vi "SSV_target_nocatch_frequency.vi"() -> ()   [LabVIEW 2014]
uses:
  <vilib>/userdefined/High Color/IMAQdx.ctl
  <vilib>/vision/driver/IMAQdx.llb/IMAQdx Acquisition Mode.ctl
  <vilib>/myRIO/Instrument Drivers/Onboard IO/PWM/typedefs/PWM Reference.ctl
  <vilib>/myRIO/Common/Instrument Driver Framework/Utilities/typedefs/myRIO Generic Hardware Reference.ctl
  <vilib>/myRIO/Common/Instrument Driver Framework/Utilities/typedefs/Hardware Version Enum.ctl
  <vilib>/myRIO/Common/Instrument Driver Framework/Utilities/typedefs/myRIO v1.0 Reference.ctl
  <vilib>/myRIO/Common/Instrument Driver Framework/Utilities/typedefs/Generic FPGA Reference.ctl
  <vilib>/myRIO/Common/Instrument Driver Framework/myRIO v1.0/PWM/typedefs/PWM Channels Enum.ctl
  <vilib>/myRIO/Instrument Drivers/Onboard IO/PWM/typedefs/PWM Configuration.ctl
  <vilib>/userdefined/High Color/nirio_resource_hc.ctl
  <vilib>/myRIO/Instrument Drivers/Onboard IO/DIO/typedefs/DIO Reference.ctl
  <vilib>/myRIO/Common/Instrument Driver Framework/myRIO v1.0/DIO/typedefs/DIO Channels List.ctl
  <vilib>/myRIO/Common/Instrument Driver Framework/myRIO v1.0/DIO/typedefs/DIO Channels Enum.ctl
  <vilib>/vision/driver/IMAQdx.llb/IMAQdx Buffer Number Mode.ctl
  <vilib>/myRIO/Common/Instrument Driver Framework/myRIO v1.0/PWM/vis/myRIO v1.1 Open PWM.vi
  <vilib>/myRIO/Common/Instrument Driver Framework/myRIO v1.0/DIO/vis/myRIO v1.1 Open DIO.vi
  <vilib>/myRIO/Common/Instrument Driver Framework/Utilities/vis/Is FPGA Ref Available.vi
  <vilib>/myRIO/Instrument Drivers/Onboard IO/DIO/vis/Read.vi
  <vilib>/Analysis/baseanly.llb/Mean (DBL).vi
  <vilib>/myRIO/Common/Instrument Driver Framework/Utilities/vis/Validate Channels.vi
  <vilib>/myRIO/Common/Instrument Driver Framework/myRIO v1.0/PWM/vis/myRIO v1.0 Reserve PWM.vi
  <vilib>/myRIO/Common/Instrument Driver Framework/myRIO v1.0/DIO/vis/myRIO v1.0 Reserve DIO.vi
  <vilib>/myRIO/Common/Instrument Driver Framework/myRIO v1.0/DIO/vis/myRIO v1.0 Close DIO.vi
  <vilib>/myRIO/Common/Instrument Driver Framework/myRIO v1.0/PWM/vis/myRIO v1.0 Close PWM.vi
  <vilib>/myRIO/Common/Instrument Driver Framework/myRIO v1.0/PWM/vis/myRIO v1.0 Build MUX Configuration PWM.vi
  <vilib>/myRIO/Common/Instrument Driver Framework/myRIO v1.0/Resource Manager/vis/myRIO v1.0 Reserve Channel List.vi
  <vilib>/myRIO/Common/Instrument Driver Framework/myRIO v1.0/DIO/vis/myRIO v1.0 Build MUX Configuration DIO.vi
  <vilib>/myRIO/Common/Instrument Driver Framework/myRIO v1.0/DIO/vis/myRIO v1.0 Unreserve DIO.vi
  <vilib>/myRIO/Common/Instrument Driver Framework/myRIO v1.0/PWM/vis/myRIO v1.0 Unreserve PWM.vi
  <vilib>/myRIO/Common/Instrument Driver Framework/myRIO v1.0/Resource Manager/vis/myRIO v1.0 Create Configuration List.vi
  <vilib>/myRIO/Common/Instrument Driver Framework/myRIO v1.0/Resource Manager/vis/myRIO v1.0 Reserve Channel.vi
  <vilib>/myRIO/Common/Instrument Driver Framework/myRIO v1.0/Resource Manager/vis/myRIO v1.0 Unreserve Channel.vi
  <vilib>/myRIO/Common/Instrument Driver Framework/myRIO v1.0/Resource Manager/vis/myRIO v1.0 Unreserve Channel List.vi
  <vilib>/myRIO/Common/Instrument Driver Framework/myRIO v1.0/Resource Manager/vis/myRIO v1.0 Build Mutex Name.vi
  <vilib>/Utility/VariantDataType/GetNumericInfo.vi
  <vilib>/Utility/error.llb/Error Cluster From Error Code.vi
  <vilib>/myRIO/Common/Instrument Driver Framework/myRIO v1.0/myRIO v1.1 Open.vi
  <vilib>/myRIO/Common/Instrument Driver Framework/Utilities/vis/IO Manager.vi
  <vilib>/myRIO/Common/Instrument Driver Framework/Utilities/vis/Configuration Manager.vi
  <vilib>/myRIO/Common/Instrument Driver Framework/myRIO v1.0/Resource Manager/vis/myRIO v1.0 Configure IO.vi
  <vilib>/myRIO/Common/Instrument Driver Framework/myRIO v1.0/myRIO v1.0 Close.vi
  <vilib>/myRIO/Common/Instrument Driver Framework/myRIO v1.0/DIO/vis/myRIO v1.0 Write DIO.vi
  <vilib>/myRIO/Common/Instrument Driver Framework/myRIO v1.0/PWM/vis/myRIO v1.0 Write PWM.vi
  <vilib>/myRIO/Common/Instrument Driver Framework/myRIO v1.0/DIO/vis/myRIO v1.0 Read DIO.vi
  <vilib>/myRIO/Common/Instrument Driver Framework/myRIO v1.0/DIO/vis/myRIO v1.0 Shutdown DIO.vi
  <vilib>/myRIO/Common/Instrument Driver Framework/myRIO v1.0/PWM/vis/myRIO v1.0 Shutdown PWM.vi
  <vilib>/myRIO/Instrument Drivers/Onboard IO/DIO/vis/myRIO DIO Open.xnode
  <vilib>/myRIO/Instrument Drivers/Onboard IO/PWM/vis/myRIO PWM Open.xnode
  <vilib>/myRIO/Express VI/Onboard Devices/LED/LED Express VI.xnode
  <vilib>/myRIO/Express VI/Onboard Devices/Button/Button Express VI.xnode
  <vilib>/vision/driver/NI_Vision_Acquisition_Software.lvlib
  <vilib>/vision/NI_Vision_Development_Module.lvlib
  <vilib>/Analysis/NI_AALBase.lvlib
  <resource>/objmgr/imaqdx.rc
  <vilib>/myRIO/Instrument Drivers/Onboard IO/DIO/DIO.lvlib
  <vilib>/myRIO/Instrument Drivers/Onboard IO/PWM/PWM.lvlib
panel:
  in  "V":cluster{dbl, dbl}(slide)={0.0, 2.8282828282828283} scale=0.0..255.0
  in  "S":cluster{dbl, dbl}(slide)={0.0, 2.8282828282828283} scale=0.0..255.0
  in  "H":cluster{dbl, dbl}(slide)={0.0, 2.8282828282828283} scale=0.0..255.0
  out "PWM Error":errorcluster
  out "Array 5":bool[](array[boolean])
  out "Array 4":bool[](array[boolean])
  out "Array 3":bool[](array[boolean])
  out "Array 2":bool[](array[boolean])
  out "Motors":bool[](array[boolean])
  in  "Min Period (ms)":dbl=500.0 format="%#_13g"
  in  "Max Period (ms)":dbl=500.0 format="%#_13g"
  out "y":dbl
  out "x":dbl
  out "Tracking Image":T1(plugin-control)
  out "Distance (in)":dbl
  in  "Diameter of Ball (in)":dbl
  out "DIO Error":errorcluster
  in  "Max Distance (in)":dbl=500.0 format="%#_13g"
  out "Camera Error":errorcluster
  out "FPS":dbl
  out "Original Image":T1(plugin-control)
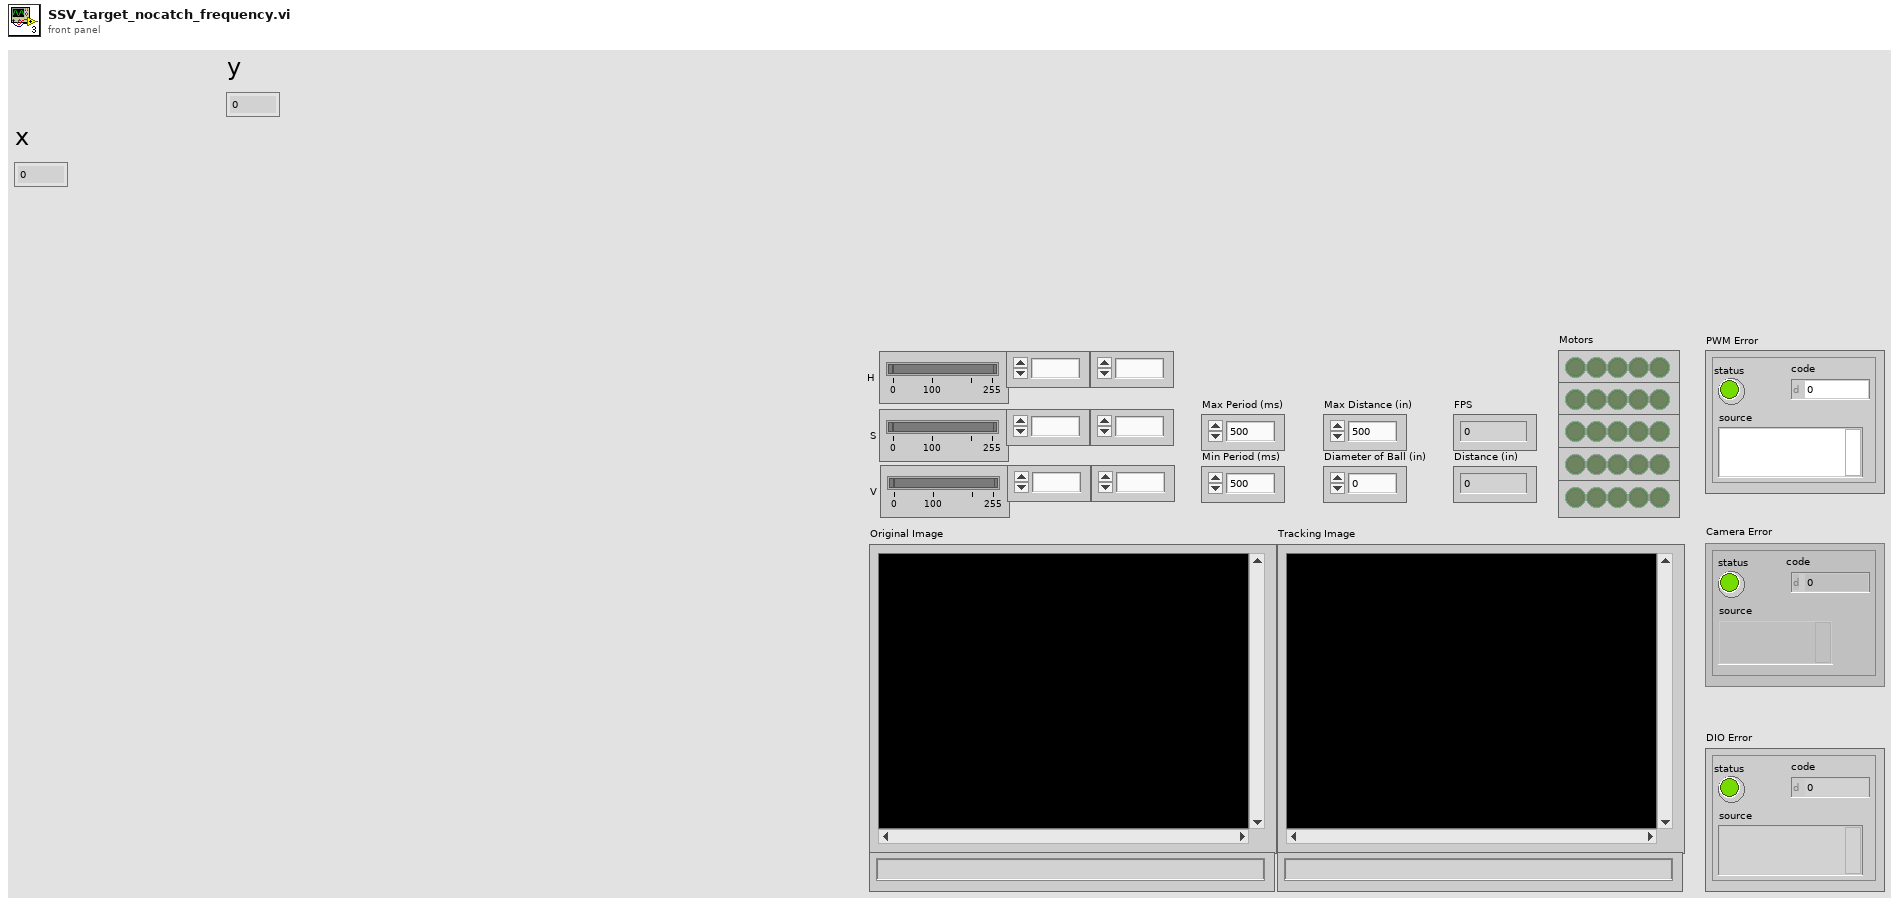
[diagram p1: front panel]
types:
  T1 = typedef "IMAQ Image.ctl" = refnum<image>
  T2 = typedef "NI_Vision_Acquisition_Software.lvlib/IMAQdx Acquisition Mode.ctl" = enum32{"One Shot", "Continuous"}
  T3 = typedef "IMAQdx.ctl" = refnum<k21>
  T4 = typedef "DIO.lvlib/DIO Reference.ctl" = cluster{"myRIO Reference":T5, "DIO Channels List":T9}
  T5 = typedef "myRIO Generic Hardware Reference.ctl" = cluster{"myRIO Model":T6, "myRIO Hardware Reference":T7}
  T6 = typedef "Hardware Version Enum.ctl" = enum16{"Unknown", "myRIO-1900", "myRIO-1950"}
  T7 = typedef "myRIO v1.0 Reference.ctl" = cluster{"Generic FPGA Reference":T8, "Allow multiple opens":bool}
  T8 = typedef "Generic FPGA Reference.ctl" = refnum<k20>
  T9 = typedef "DIO Channels List.ctl" = T10[]
  T10 = typedef "DIO Channels Enum.ctl" = enum16{"Not Connected", "C/DIO0", "C/DIO1", "C/DIO2", "C/DIO3", "C/DIO4", "C/DIO5", "C/DIO6", "C/DIO7", "A/DIO0", "A/DIO1", "A/DIO2", "A/DIO3", "A/DIO4", "A/DIO5", "A/DIO6", "A/DIO7", "A/DIO8", "A/DIO9", "A/DIO10", "A/DIO11", "A/DIO12", "A/DIO13", "A/DIO14", "A/DIO15", "B/DIO0", "B/DIO1", "B/DIO2", "B/DIO3", "B/DIO4", "B/DIO5", "B/DIO6", "B/DIO7", "B/DIO8", "B/DIO9", "B/DIO10", "B/DIO11", "B/DIO12", "B/DIO13", "B/DIO14", "B/DIO15", "LED0", "LED1", "LED2", "LED3", "Button0"}
  T11 = typedef "PWM.lvlib/PWM Reference.ctl" = cluster{"myRIO Reference":T5, "PWM Channels Enum":T12, "PWM Configuration":T13}
  T12 = typedef "PWM Channels Enum.ctl" = enum16{"Not Connected", "C/PWM0", "C/PWM1", "A/PWM0", "A/PWM1", "A/PWM2", "B/PWM0", "B/PWM1", "B/PWM2"}
  T13 = typedef "PWM.lvlib/PWM Configuration.ctl" = cluster{"Frequency":dbl, "Duty Cycle":dbl}
  T14 = typedef "nirio_resource_hc.ctl" = tag
  T15 = typedef "NI_Vision_Acquisition_Software.lvlib/IMAQdx Buffer Number Mode.ctl" = enum32{"Next", "Last", "Buffer Number"}
  T16 = typedef "Particle Parameters" = i32
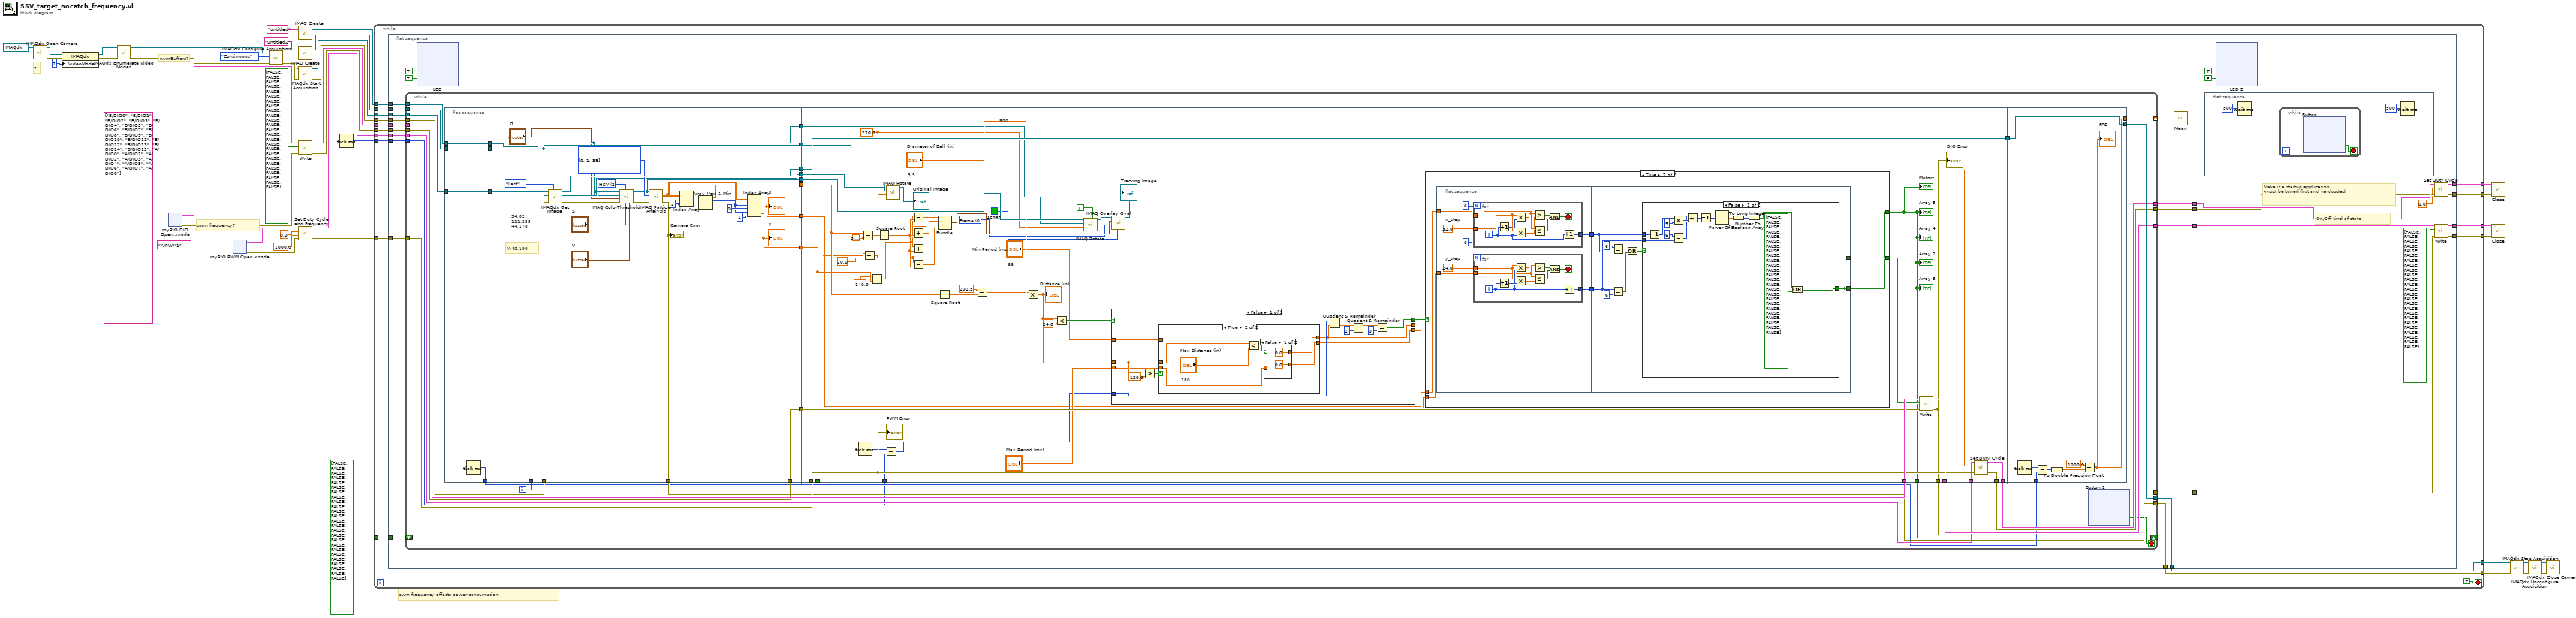
[diagram p0: block diagram]
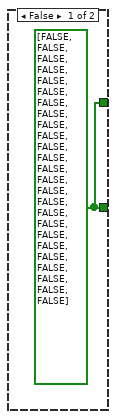
[diagram p2: hidden frame]
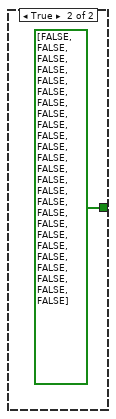
[diagram p3: hidden frame]
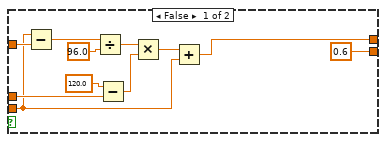
[diagram p4: hidden frame]
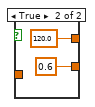
[diagram p5: hidden frame]
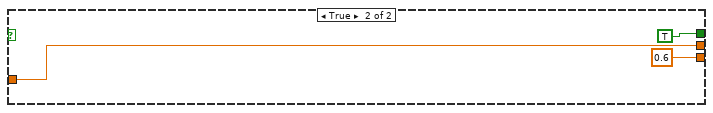
[diagram p6: hidden frame]
diagram:
  # "7"
  # "pwm frequency?"
  # "numBuffers?"
  # "pwm frequency affects power consumption"
  n1 = call <vilib>:"IMAQdx Open Camera.vi"("Session In"=T3 "cam1") -> ("error out"=w35:errorcluster, "Session Out"=w26:T3)  [unwired: 9 in]
  n2 = property class="IMAQdx"(reference=w26, error in=w35, "VideoMode"=u32 7) -> (reference out=w37:T3, error out=w39:errorcluster)
  n3 = call <vilib>:"IMAQdx Enumerate Video Modes.vi"("error in"=w39, "Session In"=w37) -> ("error out"=w40:errorcluster, "Session Out"=w38:T3)  [unwired: 6 in, 2 out]
  n4 = xnode "myRIO DIO Open.xnode"("Channel Names"=tag[] ["B/DIO0", "B/DIO1", "B/DIO2", "B/DIO3", "B/DIO4", "B/DIO5", "B/DIO6", "B/DIO7", "B/DIO8", "B/DIO9", "B/DIO10", "B/DIO11", "B/DIO12", "B/DIO13", "B/DIO14", "B/DIO15", "A/DIO0", "A/DIO1", "A/DIO2", "A/DIO3", "A/DIO4", "A/DIO5", "A/DIO6", "A/DIO7", "A/DIO8"]) -> ("error out"=w33:errorcluster, "DIO Ref Out"=w34:T4)  [unwired: 2 in]
  n5 = xnode "myRIO PWM Open.xnode"("Channel Name"=tag "A/PWM1") -> ("error out"=w30:errorcluster, "PWM Ref Out"=w29:T11)  [unwired: 2 in]
  n6 = call <vilib>:"IMAQdx Configure Acquisition.vi"("error in"=w40, "Continuous?"=IMAQdx_Acquisition_Mode."Continuous", "Session In"=w38) -> ("error out"=w36:errorcluster, "Session Out"=w24:T3)  [unwired: 7 in]
  n7 = call "IMAQ Create"("Image Name"="untitled") -> ("New Image"=w15:T1)  [unwired: 4 in, 1 out]
  n8 = call "IMAQ Create"("Image Name"="untitled2") -> ("New Image"=w19:T1)  [unwired: 4 in, 1 out]
  n9 = call <vilib>:"IMAQdx Start Acquisition.vi"("error in"=w36, "Session In"=w24) -> ("error out"=w16:errorcluster, "Session Out"=w17:T3)  [unwired: 8 in]
  n10 = call <vilib>:"Write.vi"("error in (no error)"=w33, "Values"=bool[] [FALSE, FALSE, FALSE, FALSE, FALSE, FALSE, FALSE, FALSE, FALSE, FALSE, FALSE, FALSE, FALSE, FALSE, FALSE, FALSE, FALSE, FALSE, FALSE, FALSE, FALSE, FALSE, FALSE, FALSE, FALSE], "DIO Ref In"=w34) -> ("error out"=w11:errorcluster, "DIO Ref Out"=w12:T4)  [unwired: 6 in]
  n11 = call <vilib>:"Set Duty Cycle and Frequency.vi"("error in (no error)"=w30, "Frequency [Hz]"=1000.0, "Duty Cycle"=0.0, "PWM Ref In"=w29) -> ("error out"=w13:errorcluster, "PWM Ref Out"=w14:T11)  [unwired: 5 in]
  n12 = Tick Count (ms)() -> (millisecond timer value=w18:u32)
  n13 = while {
    tunnel: bool[] [FALSE, FALSE, FALSE, FALSE, FALSE, FALSE, FALSE, FALSE, FALSE, FALSE, FALSE, FALSE, FALSE, FALSE, FALSE, FALSE, FALSE, FALSE, FALSE, FALSE, FALSE, FALSE, FALSE, FALSE, FALSE] -> [w60]
    tunnel: w19 -> [w59]
    tunnel: w18 -> [w58]
    tunnel: w17 -> [w57]
    tunnel: w16 -> [w56]
    tunnel: w15 -> [w55]
    tunnel: w14 -> [w54]
    tunnel: w13 -> [w53]
    tunnel: w12 -> [w52]
    tunnel: w11 -> [w51]
    tunnel: [w50] -> w10
    tunnel: [w49] -> w9
    tunnel: [w48] -> w4
    tunnel: [w47] -> w3
    tunnel: [w44] -> w2
    tunnel: [w43] -> w1
    stop <- FALSE stop-if-true
    n14 = flat-sequence {
      tunnel: [w79] -> w62
      tunnel: [w78] -> w61
      tunnel: w60 -> [w77]
      tunnel: w59 -> [w76]
      tunnel: w58 -> [w75]
      tunnel: w57 -> [w74]
      tunnel: w56 -> [w73]
      tunnel: w55 -> [w72]
      tunnel: w54 -> [w71]
      tunnel: w53 -> [w70]
      tunnel: w52 -> [w69]
      tunnel: w51 -> [w68]
      tunnel: [w67] -> w48
      tunnel: [w66] -> w47
      tunnel: [w65] -> w46
      tunnel: [w64] -> w45
      tunnel: w62 -> [w380]
      tunnel: w61 -> [w379]
      tunnel: [w377] -> w50
      tunnel: [w376] -> w49
      tunnel: w46 -> [w374]
      tunnel: w45 -> [w373]
      tunnel: [w372] -> w44
      tunnel: [w371] -> w43
      frame #0 {
        n15 = while {
          tunnel: w72 -> [w151]
          tunnel: w74 -> [w152]
          tunnel: [w150] -> w67
          tunnel: w76 -> [w149]
          tunnel: [w144] -> w82 mode=indexing
          tunnel: w69 -> [w138]
          tunnel: w68 -> [w136]
          tunnel: [w135] -> w65
          tunnel: w71 -> [w134]
          tunnel: w70 -> [w133]
          tunnel: [w132] -> w79
          tunnel: [w131] -> w78
          tunnel: w73 -> [w130]
          tunnel: [w129] -> w66
          tunnel: [w126] -> w64
          shift-right: [w125] -> _
          shift-left: w77 -> [w124]
          tunnel: w75 -> [w123]
          i -> [w148]
          stop <- w127 stop-if-true
          n16 = flat-sequence {
            tunnel: w149 -> [w189]
            tunnel: w151 -> [w190]
            tunnel: w152 -> [w191]
            tunnel: [w191] -> w147
            tunnel: [w190] -> w146
            tunnel: [w189] -> w145
            tunnel: [w188] -> w128
            tunnel: w148 -> [_]
            tunnel: [w215] -> w143
            tunnel: w147 -> [w217]
            tunnel: w146 -> [w196]
            tunnel: w145 -> [w195]
            tunnel: [w200] -> w141
            tunnel: [w199] -> w140
            tunnel: [w198] -> w139
            tunnel: [w212] -> w137
            tunnel: w136 -> [w212]
            tunnel: w130 -> [w211]
            tunnel: [w208] -> w129
            tunnel: [w207] -> w122
            tunnel: [w197] -> w121
            tunnel: [w196] -> w120
            tunnel: [w195] -> w119
            tunnel: w143 -> [w268]
            tunnel: [w268] -> w142
            tunnel: w141 -> [w220]
            tunnel: w140 -> [w225]
            tunnel: w139 -> [w223]
            tunnel: w138 -> [w265]
            tunnel: w137 -> [w264]
            tunnel: [w263] -> w135
            tunnel: w134 -> [w262]
            tunnel: w133 -> [w261]
            tunnel: [w260] -> w132
            tunnel: [w259] -> w131
            tunnel: [w258] -> w126
            tunnel: [w235] -> w125
            tunnel: w124 -> [_]
            tunnel: w123 -> [w245]
            tunnel: w122 -> [w234]
            tunnel: w121 -> [w237]
            tunnel: w120 -> [w233]
            tunnel: w119 -> [w238]
            tunnel: [w370] -> w150
            tunnel: w142 -> [w370]
            tunnel: w128 -> [w368]
            tunnel: [w364] -> w144
            frame #0 {
              n17 = Tick Count (ms)() -> (millisecond timer value=w188:u32)
            }
            frame #1 {
              w214 = T16[] [0, 1, 38] items=["Center of Mass X", "Center of Mass Y", "First Pixel X", "First Pixel Y", "Bounding Rect Left", "Bounding Rect Top", "Bounding Rect Right", "Bounding Rect Bottom", "Max Feret Diameter Start X", "Max Feret Diameter Start Y", "Max Feret Diameter End X", "Max Feret Diameter End Y", "Max Horiz. Segment Length Left", "Max Horiz. Segment Length Right", "Max Horiz. Segment Length Row", "-", "Bounding Rect Width", "Bounding Rect Height", "Bounding Rect Diagonal", "Perimeter", "Convex Hull Perimeter", "Holes' Perimeter", "Max Feret Diameter", "Equivalent Ellipse Major Axis", "Equivalent Ellipse Minor Axis", "Equivalent Ellipse Minor Axis (Feret)", "Equivalent Rect Long Side", "Equivalent Rect Short Side", "Equivalent Rect Diagonal", "Equivalent Rect Short Side (Feret)", "Average Horiz. Segment Length", "Average Vert. Segment Length", "Hydraulic Radius", "Waddel Disk Diameter", "-", "Area", "Holes' Area", "Particle & Holes' Area", "Convex Hull Area", "Image Area", "-", "Number of Holes", "Number of Horiz. Segments", "Number of Vert. Segments", "-", "Orientation", "Max Feret Diameter Orientation", "-", "% Area/Image Area", "% Area/(Particle & Holes' Area)", "Ratio of Equivalent Ellipse Axes", "Ratio of Equivalent Rect Sides", "-", "Elongation Factor", "Compactness Factor", "Heywood Circularity Factor", "Type Factor", "-", "Sum X", "Sum Y", "Sum XX", "Sum XY", "Sum YY", "Sum XXX", "Sum XXY", "Sum XYY", "Sum YYY", "-", "Moment of Inertia XX", "Moment of Inertia XY", "Moment of Inertia YY", "Moment of Inertia XXX", "Moment of Inertia XXY", "Moment of Inertia XYY", "Moment of Inertia YYY", "Norm. Moment of Inertia XX", "Norm. Moment of Inertia XY", "Norm. Moment of Inertia YY", "Norm. Moment of Inertia XXX", "Norm. Moment of Inertia XXY", "Norm. Moment of Inertia XYY", "Norm. Moment of Inertia YYY", "Hu Moment 1", "Hu Moment 2", "Hu Moment 3", "Hu Moment 4", "Hu Moment 5", "Hu Moment 6", "Hu Moment 7"] ("Pixel Measurements")
              w216 = u16 2 items=["RGB", "HSL", "HSV", "HSI"] ("Color Mode")
              # "V:40,190"
              # "54,82\n111,255\n44,178"
              n18 = call <vilib>:"IMAQdx Get Image.vi"("Buffer Number Mode (Next)"=IMAQdx_Buffer_Number_Mode."Last" ("Buffer Number Mode"), "error in"=w211, "Image In"=w195, "Session In"=w217) -> ("error out"=w210:errorcluster, "Image Out"=w197:T1, "Session Out"=w215:T3)  [unwired: 4 in, 1 out]
              n19 = call "IMAQ ColorThreshold"("Blue or Luma or Val or Inten Range"="V", "Green or Sat Range"="S", "Color Mode"=w216, "error in (no error)"=w210, "Red or Hue Range"="H", "Image Dst"=w196, "Image Src"=w197) -> ("error out"=w209:errorcluster, "Image Dst Out"=w207:T1)  [unwired: 3 in]
              n20 = call "IMAQ Particle Analysis"("error in (no error)"=w209, "Pixel Measurements"=w214, "Image"=w207) -> ("error out"=w208:errorcluster, "Particle Measurements (Pixels)"=w201:dbl[][])  [unwired: 3 in, 4 out]
              "Camera Error" <- w208
              n21 = Index Array(array=w201, index (col)=2 ("disabled index (col)")) -> (element=w203:dbl[])  [unwired: 1 in]
              n22 = Array Max & Min(array=w203) -> (max value=w198:dbl, max index (indices)=w204:i32)  [unwired: 2 out]
              n23 = Index Array(array=w201, index (row) #1=w204, index (col) #1=0 ("disabled index (col)"), index (row) #2=w204, index (col) #2=1 ("disabled index (col)")) -> (element #1=w200:dbl, element #2=w199:dbl)
              "x" <- w200
              "y" <- w199
            }
            frame #2 {
              w232 = sgl 270.0 ("Angle (degrees)")
              w229 = u32 0 items=["Frame", "Fill"] ("Drawing Mode (Frame)")
              # "3.5"
              # "500"
              # "66"
              n24 = Tick Count (ms)() -> (millisecond timer value=w246:u32)
              n25 = Divide(x=w223, y=3.141592653589793) -> (x/y=w247:dbl)
              n26 = Subtract(x=w220, y=20.0 ("y 2")) -> (x-y=w218:dbl)
              n27 = Subtract(x=140.0 ("x 3"), y=w225) -> (x-y=w221:dbl)
              n28 = Square Root(x=w247) -> (sqrt(x)=w222:dbl)
              n29 = Subtract(x=w246, y=w245) -> (x-y=w242:u32)
              n30 = call "IMAQ Rotate"("Angle (degrees)"=w232, "Image Dst"=w238, "Image Src"=w237) -> ("Image Dst Out"=→"Original Image":T1)  [unwired: 7 in, 1 out]
              n31 = Subtract(x=w221, y=w222) -> (x-y=w252:dbl)
              n32 = Add(x=w218, y=w222) -> (x+y=w251:dbl)
              n33 = Add(x=w221, y=w222) -> (x+y=w250:dbl)
              n34 = Subtract(x=w218, y=w222) -> (x-y=w249:dbl)
              n35 = Bundle(w252, w251, w250, w249) -> (w230:cluster{dbl, dbl, dbl, dbl})  [unwired: 1 in]
              n36 = Square Root(x=w223) -> (sqrt(x)=w255:dbl)
              n37 = Divide(x=202.5, y=w255) -> (x/y=w256:dbl)
              n38 = Multiply(x=w256, y="Diameter of Ball (in)") -> (x*y=w253:dbl)
              "Distance (in)" <- w253
              n39 = Less?(x=w253, y=24.0) -> (x < y?=w267:bool)
              n40 = call "IMAQ Rotate"("Maintain Size"=TRUE, "Angle (degrees)"=w232, "Image Dst"=w233, "Image Src"=w234) -> ("Image Dst Out"=w231:T1)  [unwired: 6 in, 1 out]
              n41 = call "IMAQ Overlay Oval"("Color"=u32 46081, "Drawing Mode (Frame)"=w229, "Bounding Rectangle"=w230, "Image"=w231) -> ("Image Out"=→"Tracking Image":T1)  [unwired: 6 in, 1 out]
              n42 = case shown="False" w267 {
                tunnel: w253 -> [w337 _]
                tunnel: [w329 w362] -> _
                tunnel: [w327 0.6] -> w240
                tunnel: "Max Period (ms)" -> [w336 _]
                tunnel: "Min Period (ms)" -> [w335 w362]
                tunnel: w242 -> [w330 _]
                tunnel: [w328 TRUE] -> w241
                frame False {
                  n43 = Greater?(x=w337, y=120.0) -> (0:w339:bool)
                  n44 = case shown="True" w339 {
                    tunnel: w337 -> [w349 w353]
                    tunnel: [w350 w355] -> w329
                    tunnel: [0.6 w351] -> w327
                    tunnel: w336 -> [w340 w356]
                    tunnel: w335 -> [w342 _]
                    frame False {
                      n45 = Subtract(x=w340, y=w342) -> (x-y=w341:dbl)
                      n46 = Divide(x=w341, y=96.0) -> (x/y=w347:dbl)
                      n47 = Subtract(x=120.0 ("y"), y=w349) -> (x-y=w345:dbl)
                      n48 = Multiply(x=w347, y=w345) -> (x*y=w344:dbl)
                      n49 = Add(x=w344, y=w340) -> (x+y=w350:dbl)
                    }
                    frame True {
                      # "180"
                      n50 = Less?(x=w353, y="Max Distance (in)") -> (x < y?=w354:bool)
                      n51 = case shown="False" w354 {
                        tunnel: [0.0 120.0] -> w355
                        tunnel: [0.0 0.6] -> w351
                        tunnel: w356 -> [_ _]
                        frame False {
                        }
                        frame True {
                        }
                      }
                    }
                  }
                  n52 = Quotient & Remainder(x=w330, y=w329) -> (floor(x/y)=w331:dbl)  [unwired: 1 out]
                  n53 = Quotient & Remainder(x=w331, y=u32 2) -> (x-y*floor(x/y)=w333:dbl)  [unwired: 1 out]
                  n54 = Equal?(x=w333, y=u32 0) -> (x = y?=w328:bool)
                }
                frame True {
                }
              }
              n55 = case shown="True" w241 {
                tunnel: [w269 w273] -> w236
                tunnel: [w269 w272] -> w235
                tunnel: w220 -> [_ w271]
                tunnel: w225 -> [_ w270]
                frame False {
                  w269 = bool[] [FALSE, FALSE, FALSE, FALSE, FALSE, FALSE, FALSE, FALSE, FALSE, FALSE, FALSE, FALSE, FALSE, FALSE, FALSE, FALSE, FALSE, FALSE, FALSE, FALSE, FALSE, FALSE, FALSE, FALSE, FALSE]
                }
                frame True {
                  n56 = flat-sequence {
                    tunnel: [w281] -> w275
                    tunnel: w270 -> [w277]
                    tunnel: w271 -> [w278]
                    tunnel: [w276] -> w274
                    tunnel: w275 -> [w310]
                    tunnel: [w311] -> w273
                    tunnel: [w311] -> w272
                    tunnel: w274 -> [w309]
                    frame #0 {
                      w279 = 32.0  # x_step
                      w282 = 24.0  # y_step
                      n57 = for {
                        N: 6 -> [_]
                        tunnel: w279 -> [w289]
                        tunnel: w278 -> [w291]
                        tunnel: [w284] -> w276
                        i -> [w288]
                        stop <- w285 stop-if-true
                        n58 = Increment(x=w288) -> (x+1=w287:i32)
                        n59 = Multiply(x=w289, y=w287) -> (x*y=w286:dbl)
                        n60 = Multiply(x=w289, y=w288) -> (x*y=w290:dbl)
                        n61 = Greater?(x=w291, y=w290) -> (0:w293:bool)
                        n62 = Less Or Equal?(x=w291, y=w286) -> (x <= y?=w292:bool)
                        n63 = And(x=w293, y=w292) -> (x .and. y?=w285:bool)
                        n64 = Increment(x=w288) -> (x+1=w284:i32)
                      }
                      n65 = for {
                        N: 6 -> [_]
                        tunnel: w282 -> [w299]
                        tunnel: w277 -> [w298]
                        tunnel: [w294] -> w281
                        i -> [w302]
                        stop <- w297 stop-if-true
                        n66 = Increment(x=w302) -> (x+1=w303:i32)
                        n67 = Multiply(x=w299, y=w302) -> (x*y=w295:dbl)
                        n68 = Multiply(x=w299, y=w303) -> (x*y=w296:dbl)
                        n69 = Greater?(x=w298, y=w295) -> (0:w300:bool)
                        n70 = Less Or Equal?(x=w298, y=w296) -> (x <= y?=w301:bool)
                        n71 = And(x=w300, y=w301) -> (x .and. y?=w297:bool)
                        n72 = Increment(x=w302) -> (x+1=w294:i32)
                      }
                    }
                    frame #1 {
                      n73 = Equal?(x=6, y=w309) -> (x = y?=w305:bool)
                      n74 = Equal?(x=w310, y=6) -> (x = y?=w306:bool)
                      n75 = Or(x=w305, y=w306) -> (x .or. y?=w304:bool)
                      n76 = case shown="False" w304 {
                        tunnel: [w316 bool[] [FALSE, FALSE, FALSE, FALSE, FALSE, FALSE, FALSE, FALSE, FALSE, FALSE, FALSE, FALSE, FALSE, FALSE, FALSE, FALSE, FALSE, FALSE, FALSE, FALSE, FALSE, FALSE, FALSE, FALSE, FALSE]] -> w311
                        tunnel: w310 -> [w314 _]
                        tunnel: w309 -> [w312 _]
                        frame False {
                          n77 = Decrement(x=w312) -> (x-1=w324:i32)
                          n78 = Multiply(x=w324, y=5) -> (x*y=w319:i32)
                          n79 = Subtract(x=6, y=w314) -> (x-y=w313:i32)
                          n80 = Add(x=w313, y=w319) -> (x+y=w323:i32)
                          n81 = Decrement(x=w323) -> (x-1=w320:i32)
                          n82 = Power Of 2(x=w320) -> (2^x=w322:dbl)
                          n83 = To Long Integer(number=w322) -> (32bit integer=w321:i32)
                          n84 = Number To Boolean Array(number=w321) -> (Boolean array=w318:bool[])
                          n85 = Or(x=w318, y=bool[] [FALSE, FALSE, FALSE, FALSE, FALSE, FALSE, FALSE, FALSE, FALSE, FALSE, FALSE, FALSE, FALSE, FALSE, FALSE, FALSE, FALSE, FALSE, FALSE, FALSE, FALSE, FALSE, FALSE, FALSE, FALSE]) -> (x .or. y?=w316:bool[])
                        }
                        frame True {
                        }
                      }
                    }
                  }
                }
              }
              "Motors" <- w235
              "Array 4" <- w235
              "Array 2" <- w235
              "Array 3" <- w235
              "Array 5" <- w235
              n86 = call <vilib>:"Write.vi"("error in (no error)"=w264, "Values"=w236, "DIO Ref In"=w265) -> ("error out"=w258:errorcluster, "DIO Ref Out"=w263:T4)  [unwired: 6 in]
              "DIO Error" <- w258
              n87 = call <vilib>:"Set Duty Cycle.vi"("error in (no error)"=w261, "Duty Cycle"=w240, "PWM Ref In"=w262) -> ("error out"=w259:errorcluster, "PWM Ref Out"=w260:T11)  [unwired: 6 in]
              "PWM Error" <- w261
            }
            frame #3 {
              n88 = Tick Count (ms)() -> (millisecond timer value=w369:u32)
              n89 = Subtract(x=w369, y=w368) -> (x-y=w367:u32)
              n90 = To Double Precision Float(number=w367) -> (double precision float=w366:dbl)
              n91 = Divide(x=1000.0, y=w366) -> (x/y=w364:dbl)
              "FPS" <- w364
            }
          }
          n92 = xnode "Button 2"() -> ("Value"=w127:bool)  [unwired: 1 in, 1 out]
        }
        n93 = xnode "LED"("LED0"=TRUE, "LED1"=TRUE) -> ()  [unwired: 1 in, 1 out]
        n94 = call-poly <vilib>:"Mean.vi"("X"=w82) -> ()  [unwired: 2 out]
      }
      frame #1 {
        # "Make it a startup application\n-must be tuned first and hardcoded"
        # "On/Off kind of state"
        n95 = flat-sequence {
          frame #0 {
            n96 = Wait (ms)(milliseconds to wait=u32 500) -> ()  [unwired: 1 out]
          }
          frame #1 {
            n97 = while {
              stop <- w384 stop-if-true
              n98 = xnode "Button"() -> ("Value"=w384:bool)  [unwired: 1 in, 1 out]
            }
          }
          frame #2 {
            n99 = Wait (ms)(milliseconds to wait=u32 500) -> ()  [unwired: 1 out]
          }
        }
        n100 = xnode "LED 2"("LED0"=TRUE, "LED1"=FALSE) -> ()  [unwired: 1 in, 1 out]
        n101 = call <vilib>:"Set Duty Cycle.vi"("error in (no error)"=w379, "Duty Cycle"=0.0, "PWM Ref In"=w380) -> ("error out"=w376:errorcluster, "PWM Ref Out"=w377:T11)  [unwired: 6 in]
        n102 = call <vilib>:"Write.vi"("error in (no error)"=w373, "Values"=bool[] [FALSE, FALSE, FALSE, FALSE, FALSE, FALSE, FALSE, FALSE, FALSE, FALSE, FALSE, FALSE, FALSE, FALSE, FALSE, FALSE, FALSE, FALSE, FALSE, FALSE, FALSE, FALSE, FALSE, FALSE, FALSE], "DIO Ref In"=w374) -> ("error out"=w371:errorcluster, "DIO Ref Out"=w372:T4)  [unwired: 6 in]
      }
    }
  }
  n103 = call <vilib>:"Close.vi"("error in (no error)"=w9, "PWM Ref In"=w10) -> ()  [unwired: 9 in, 1 out]
  n104 = call <vilib>:"Close.vi"("error in (no error)"=w1, "DIO Ref In"=w2) -> ()  [unwired: 9 in, 1 out]
  n105 = call <vilib>:"IMAQdx Stop Acquisition.vi"("error in"=w3, "Session In"=w4) -> ("error out"=w7:errorcluster, "Session Out"=w5:T3)  [unwired: 8 in]
  n106 = call <vilib>:"IMAQdx Unconfigure Acquisition.vi"("error in"=w7, "Session In"=w5) -> ("error out"=w8:errorcluster, "Session Out"=w6:T3)  [unwired: 8 in]
  n107 = call <vilib>:"IMAQdx Close Camera.vi"("error in"=w8, "Session In"=w6) -> ()  [unwired: 9 in, 1 out]
